vi "Case blocks.vi"() -> ()   [LabVIEW 2024]
panel:
  out "Numeric 4":dbl
  in  "Numeric 3":dbl
  in  "Numeric 2":i32
  in  "Numeric":dbl
  out "true":bool
  in  "Boolean":bool
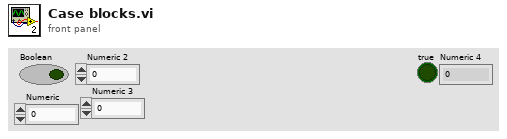
[diagram p1: front panel]
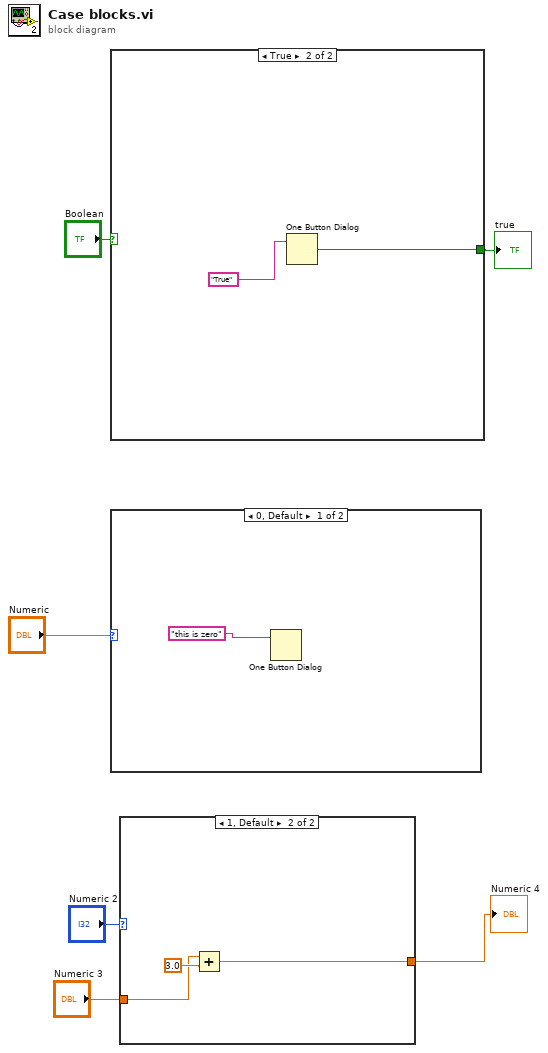
[diagram p0: block diagram]
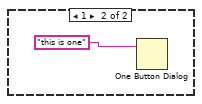
[diagram p3: hidden frame]
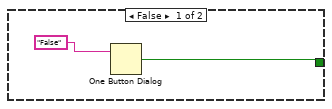
[diagram p4: hidden frame]
diagram:
  n1 = case shown="True" "Boolean" {
    tunnel: [w7 w9] -> w5
    frame False {
      n2 = One Button Dialog(message="False") -> (true=w7:bool)  [unwired: 1 in]
    }
    frame True {
      n3 = One Button Dialog(message="True") -> (true=w9:bool)  [unwired: 1 in]
    }
  }
  "true" <- w5
  n4 = case shown="0, Default" "Numeric" {
    frame 0, Default {
      n5 = One Button Dialog(message="this is zero") -> ()  [unwired: 1 in, 1 out]
    }
    frame 1 {
      n6 = One Button Dialog(message="this is one") -> ()  [unwired: 1 in, 1 out]
    }
  }
  n7 = case shown="1, Default" "Numeric 2" {
    tunnel: "Numeric 3" -> [_ w13]
    tunnel: [_ w15] -> w1
    frame 0 {
    }
    frame 1, Default {
      n8 = Add(x=w13, y=3.0) -> (x+y=w15:dbl)
    }
  }
  "Numeric 4" <- w1
